vi "PumpAcid.vi"(8 "error in":errorcluster, 11 "VISA resource name":refnum<visa-resource-name>="ASRL2::INSTR") -> (0 "error out":errorcluster, 3 "VISA resource out":refnum<visa-resource-name>="ASRL2::INSTR")   [LabVIEW 2010]
panel:
  in  "Action 2":u8(ring) items=["TurnON_1"=8, "TurnON_PUMP"=9, "TurnON_3"=10, "TurnON_4"=11, "TurnOFF_1"=0, "TurnOFF_PUMP"=1, "TurnOFF_3"=2, "TurnOFF_4"=3, "OpenAll"=30, "CloseAllRelay"=29]
  in  "Action":u8(ring) items=["TurnON_1"=8, "TurnON_PUMP"=9, "TurnON_3"=10, "TurnON_4"=11, "TurnOFF_1"=0, "TurnOFF_PUMP"=1, "TurnOFF_3"=2, "TurnOFF_4"=3, "OpenAll"=30, "CloseAllRelay"=29]
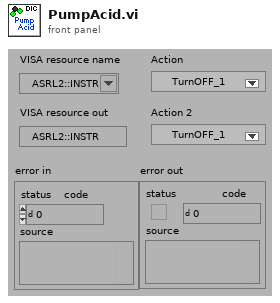
[diagram p1: front panel]
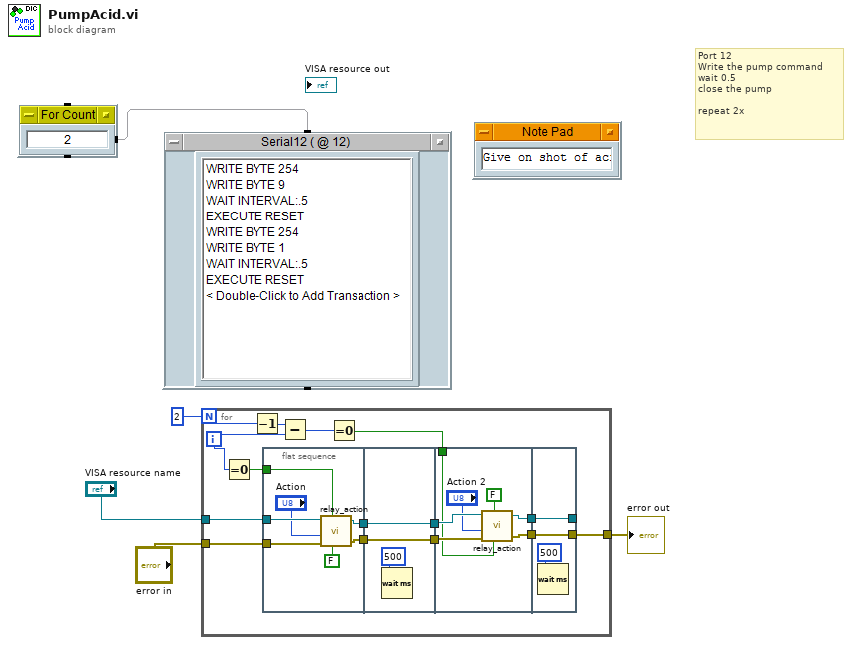
[diagram p0: block diagram]
diagram:
  # "Port 12\nWrite the pump command \nwait 0.5 \nclose the pump\n\nrepeat 2x"
  n1 = for {
    N: 2 -> [w12]
    tunnel: "VISA resource name" -> [w18]
    tunnel: "error in" -> [w17]
    tunnel: [w5] -> w1
    i -> [w10]
    n2 = Equal To 0?(x=w10) -> (x = 0?=w19:bool)
    n3 = Decrement(x=w12) -> (x-1=w11:i32)
    n4 = flat-sequence {
      tunnel: w19 -> [w26]
      tunnel: w18 -> [w25]
      tunnel: w17 -> [w24]
      tunnel: [w22] -> w15
      tunnel: [w21] -> w13
      tunnel: [w28] -> w16
      tunnel: w15 -> [w28]
      tunnel: [w27] -> w14
      tunnel: w13 -> [w27]
      tunnel: w16 -> [w34]
      tunnel: w14 -> [w36]
      tunnel: w8 -> [w32]
      tunnel: [w31] -> w7
      tunnel: [w30] -> w6
      tunnel: [w38] -> w5
      tunnel: [w39] -> _
      tunnel: w7 -> [w39]
      tunnel: w6 -> [w38]
      frame #0 {
        n5 = call "relay_action.vi"("VISA resource name"=w25, "init?"=w26, "Action"="Action", "Quit?"=FALSE, "error in"=w24) -> ("VISA resource name 2"=w22:refnum<visa-resource-name>, "error out"=w21:errorcluster)  [unwired: 2 in]
      }
      frame #1 {
        n6 = Wait (ms)(milliseconds to wait=500) -> ()  [unwired: 1 out]
      }
      frame #2 {
        n7 = call "relay_action.vi"("VISA resource name"=w34, "init?"=FALSE, "Action"="Action 2", "Quit?"=w32, "error in"=w36) -> ("VISA resource name 2"=w31:refnum<visa-resource-name>, "error out"=w30:errorcluster)  [unwired: 2 in]
      }
      frame #3 {
        n8 = Wait (ms)(milliseconds to wait=500) -> ()  [unwired: 1 out]
      }
    }
    n9 = Subtract(x=w11, y=w10) -> (x-y=w9:i32)
    n10 = Equal To 0?(x=w9) -> (x = 0?=w8:bool)
  }
  "error out" <- w1
